vi "Get illumination arm.vi"(8 "error in (no error)":errorcluster, 11 "Tomo in":refnum<class "Tomo.lvclass">) -> (0 "error out":errorcluster, 2 "Illumination arm":bool, 3 "Tomo out":refnum<class "Tomo.lvclass">)   [LabVIEW 2012, in "Tomo.lvclass"]
uses:
  Tomo.lvclass
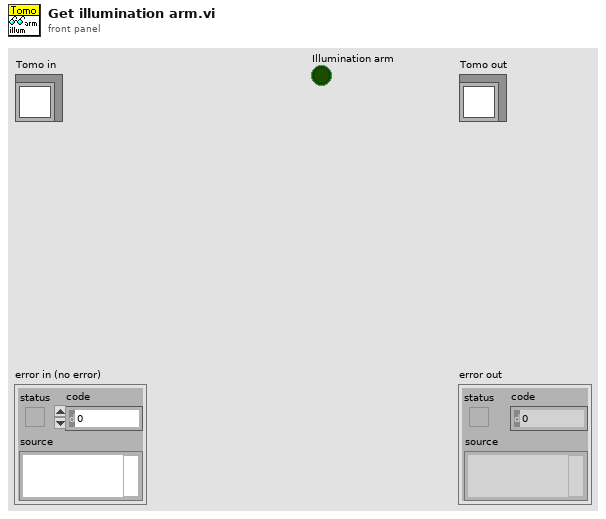
[diagram p1: front panel]
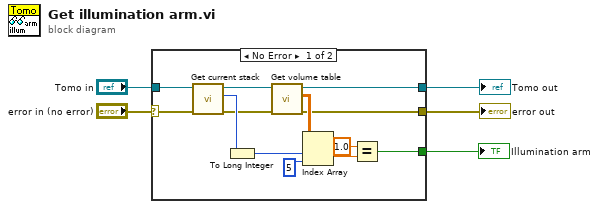
[diagram p0: block diagram]
diagram:
  n1 = case shown="No Error" "error in (no error)" {
    selector: "error in (no error)" -> [w7 w20]
    tunnel: [w6 w20] -> w4
    tunnel: [w14 w19] -> w2
    tunnel: "Tomo in" -> [w15 w19]
    tunnel: [w8 _] -> w1
    frame No Error {
      n2 = call-dynamic "Get current stack.vi"("error in (no error)"=w7, "Tomo in"=w15) -> ("error out"=w11:errorcluster, "Current stack"=w13:u16, "Tomo out"=w16:refnum<class "Tomo.lvclass">)  [unwired: 7 in]
      n3 = To Long Integer(number=w13) -> (32bit integer=w18:i32)
      n4 = call-dynamic "Get volume table.vi"("error in (no error)"=w11, "Tomo in"=w16) -> ("error out"=w6:errorcluster, "Volume table out"=w12:dbl[][], "Tomo out"=w14:refnum<class "Tomo.lvclass">)  [unwired: 7 in]
      n5 = Index Array(array=w12, index (row)=w18, index (col)=5 ("disabled index (col)")) -> (element=w10:dbl)
      n6 = Equal?(x=1.0, y=w10) -> (x = y?=w8:bool)
    }
    frame Error {
    }
  }
  "error out" <- w4
  "Tomo out" <- w2
  "Illumination arm" <- w1
